vi "Coverage Analyzer View.vi"(8 "error in (no error)":errorcluster, 11 "Code Coverage":map{path, dbl}(c390)) -> (0 "error out":errorcluster)   [LabVIEW 2020, in "Coverage Analyzer.lvclass"]
uses:
  Coverage Analyzer.lvclass
  Coverage Analyzer.lvclass/Coverage Analyzer.ctl
  <vilib>/Analysis/baseanly.llb/Mean (DBL).vi
  fde09a69-7451-4da4-9368-3dcb0be6c936.vi
  <vilib>/Comparison/Less/Less Functor/Less Functor.lvclass
  <vilib>/Analysis/NI_AALBase.lvlib
panel:
  in  "Method Test Times":i32(listbox)
  out "Debug disabled VIs":string
  out "Coverage for Executed VIs":string
  out "Fraction of VIs Executed":string
  in  "Hide VIs not executed?":bool=TRUE
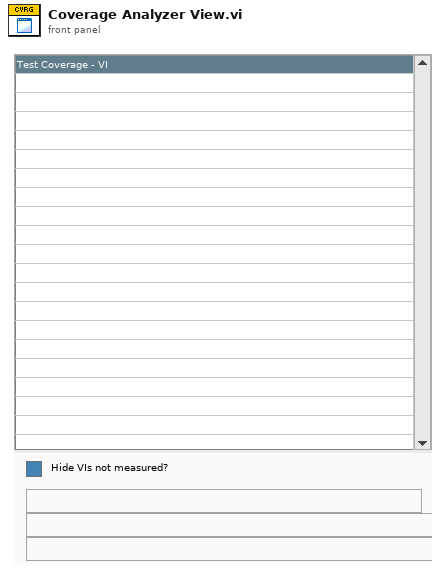
[diagram p1: front panel]
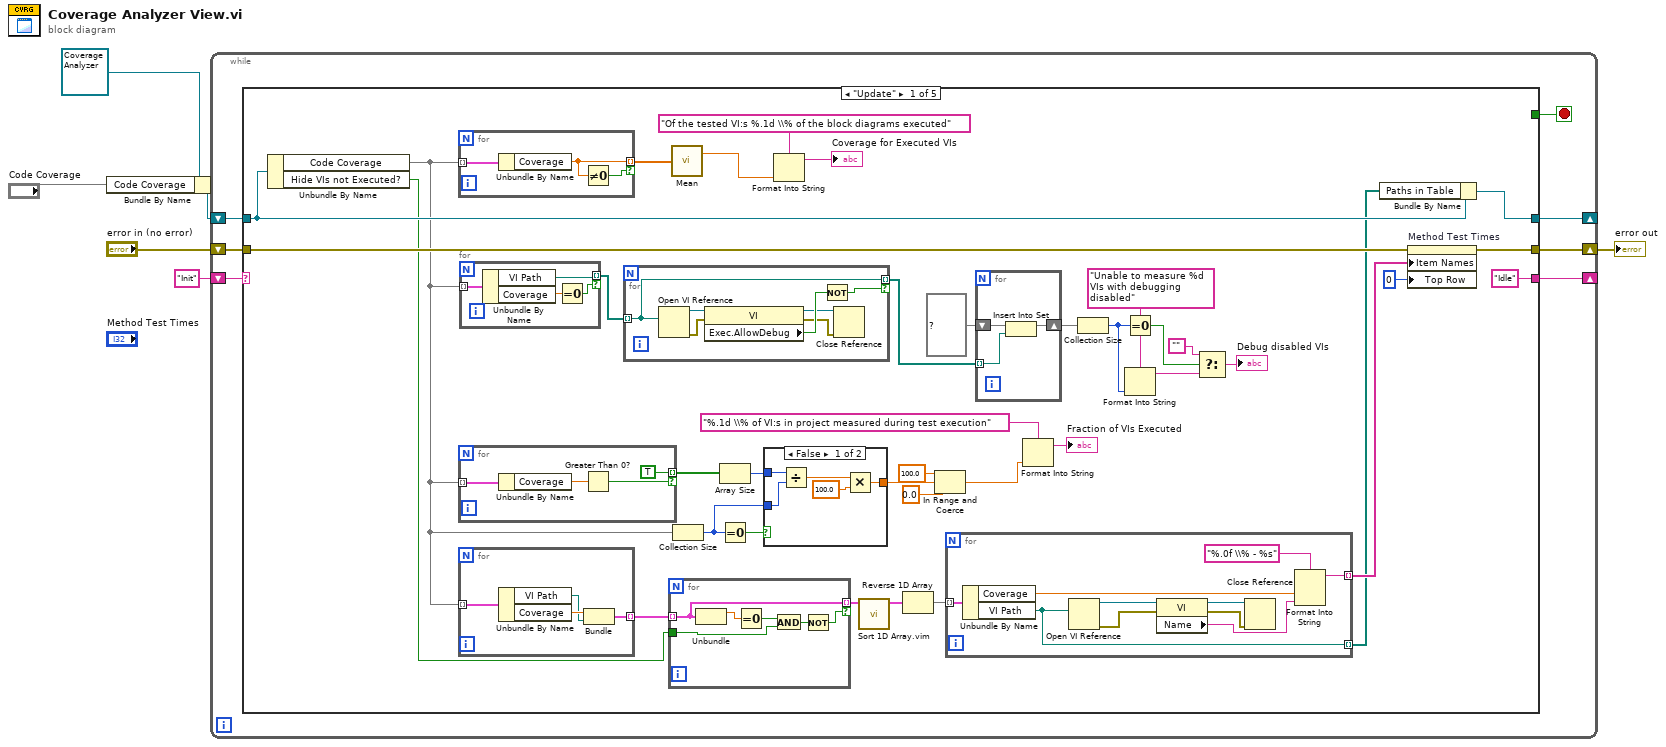
[diagram p0: block diagram]
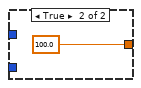
[diagram p2: hidden frame]
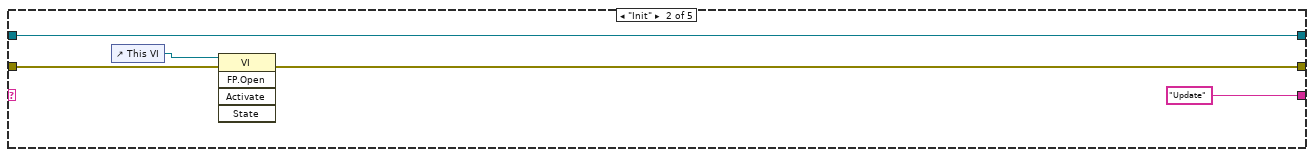
[diagram p3: hidden frame]
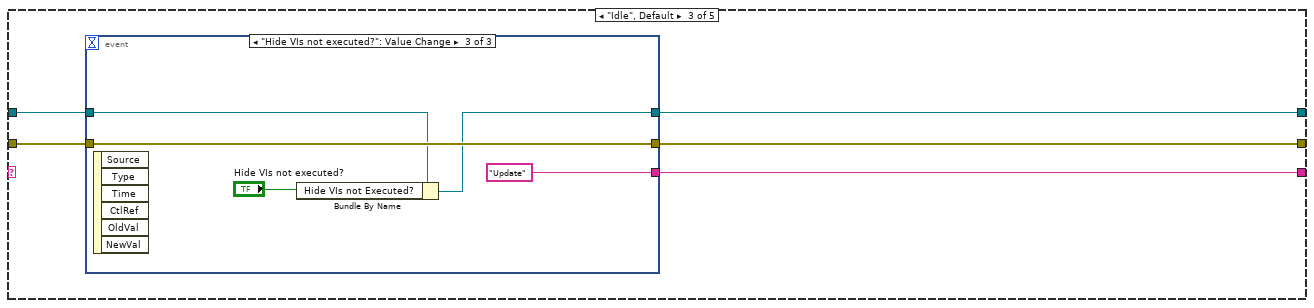
[diagram p4: hidden frame]
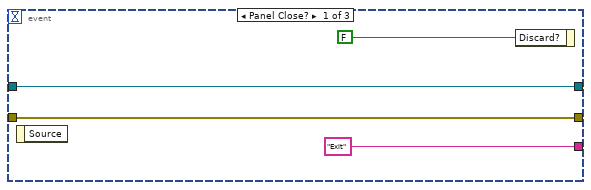
[diagram p5: hidden frame]
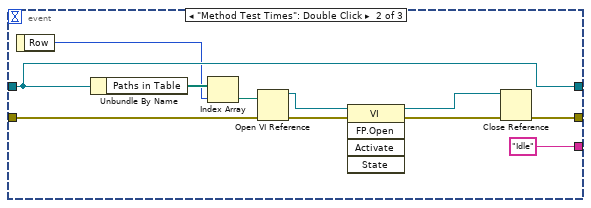
[diagram p6: hidden frame]
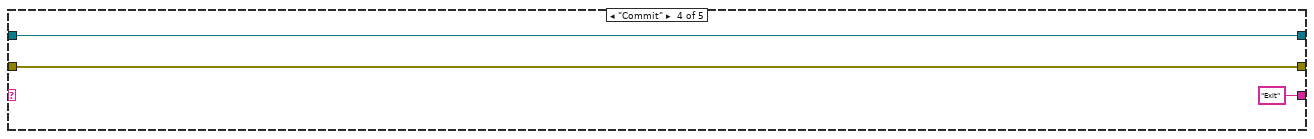
[diagram p7: hidden frame]
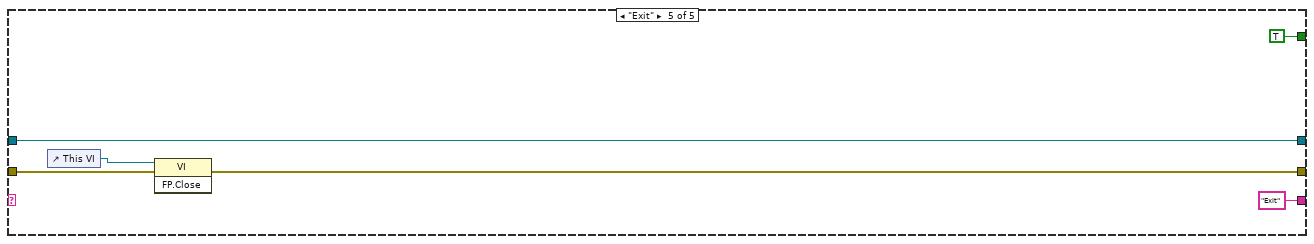
[diagram p8: hidden frame]
diagram:
  n1 = Bundle By Name(cluster=refnum<class "Coverage Analyzer.lvclass"> refnum ("Coverage Analyzer Result View.lvclass"), "Code Coverage"="Code Coverage") -> (w2:refnum<class "Coverage Analyzer.lvclass">)
  n2 = while {
    shift-right: [w10] -> _
    shift-left: w2 -> [w11]
    shift-right: [w7] -> w4
    shift-left: "error in (no error)" -> [w12]
    shift-right: [w9] -> _
    shift-left: "Init" -> [w13]
    stop <- w8 stop-if-true
    n3 = case shown="\"Update\"" w13 {
      tunnel: [w50 w101 w108 w131 w133] -> w7
      tunnel: w12 -> [w46 w100 w107 w131 w132]
      tunnel: w11 -> [w43 w99 w106 w130 w137]
      tunnel: [w48 w99 w105 w130 w137] -> w10
      tunnel: ["Idle" "Update" w104 "Exit" "Exit"] -> w9
      tunnel: [_ _ _ _ TRUE] -> w8
      frame "Update" {
        n4 = Unbundle By Name(w43) -> ("Code Coverage"=w18:map{path, dbl}, "Hide VIs not Executed?"=w17:bool)
        n5 = for {
          tunnel: w18 -> [w68] mode=indexing
          tunnel: [w67] -> w29 mode=indexing if=w66
          n6 = Unbundle By Name(w68) -> ("Coverage"=w67:dbl)
          n7 = Not Equal To 0?(x=w67) -> (x != 0?=w66:bool)
        }
        n8 = for {
          tunnel: w18 -> [w72] mode=indexing
          tunnel: [TRUE] -> w35 mode=indexing if=w69
          n9 = Unbundle By Name(w72) -> ("Coverage"=w71:dbl)
          n10 = Greater Than 0?(x=w71) -> (x > 0?=w69:bool)
        }
        n11 = for {
          tunnel: w18 -> [w88] mode=indexing
          tunnel: [w86] -> w40 mode=indexing
          n12 = Unbundle By Name(w88) -> ("VI Path"=w85:path, "Coverage"=w87:dbl)
          n13 = Bundle("Coverage"=w87, "VI Path"=w85) -> (w86:cluster{"Coverage":dbl, "VI Path":path})  [unwired: 1 in]
        }
        n14 = for {
          tunnel: w18 -> [w65] mode=indexing
          tunnel: [w62] -> w19 mode=indexing if=w63
          n15 = Unbundle By Name(w65) -> ("VI Path"=w62:path, "Coverage"=w64:dbl)
          n16 = Equal To 0?(x=w64) -> (x = 0?=w63:bool)
        }
        n17 = for {
          tunnel: w19 -> [w56] mode=indexing
          tunnel: [w56] -> w21 mode=indexing if=w55
          n18 = Open VI Reference(vi path=w56) -> (vi reference=w61:refnum<vi>, error out=w60:errorcluster)  [unwired: 5 in]
          n19 = property class="VI"(reference=w61, error in=w60) -> (reference out=w57:refnum<vi>, error out=w58:errorcluster, "Exec.AllowDebug"=w59:bool)
          n20 = Not(x=w59) -> (.not. x?=w55:bool)
          n21 = Close Reference(reference=w57, error in (no error)=w58) -> ()  [unwired: 1 out]
        }
        n22 = for {
          tunnel: [w84] -> w41 mode=indexing if=w79
          tunnel: w40 -> [w84] mode=indexing
          tunnel: w17 -> [w81]
          n23 = Unbundle(w84) -> ("Coverage"=w83:dbl)  [unwired: 1 out]
          n24 = Equal To 0?(x=w83) -> (x = 0?=w82:bool)
          n25 = And(x=w82, y=w81) -> (x .and. y?=w80:bool)
          n26 = Not(x=w80) -> (.not. x?=w79:bool)
        }
        n27 = call-poly <vilib>:"Mean.vi"("X"=w29) -> ("mean"=w30:dbl)  [unwired: 1 out]
        n28 = Collection Size(1:w18) -> (0:w33:i32)
        n29 = Array Size(array=w35) -> (size(s)=w36:i32)
        n30 = Equal To 0?(x=w33) -> (x = 0?=w32:bool)
        n31 = case shown="False" w32 {
          tunnel: w36 -> [w77 _]
          tunnel: [w74 100.0] -> w34
          tunnel: w33 -> [w75 _]
          frame False {
            n32 = Divide(x=w77, y=w75) -> (x/y=w76:dbl)
            n33 = Multiply(x=w76, y=100.0) -> (x*y=w74:dbl)
          }
          frame True {
          }
        }
        n34 = Format Into String(format string="Of the tested VI:s %.1d \\% of the block diagrams executed", w30) -> (resulting string=→"Coverage for Executed VIs":string)  [unwired: 2 in, 1 out]
        n35 = call "Sort 1D Array.vim"("unsorted array"=w41) -> ("sorted array"=w37:cluster{"Coverage":dbl, "VI Path":path}[])  [unwired: 10 in]
        n36 = Reverse 1D Array(array=w37) -> (reversed array=w38:cluster{"Coverage":dbl, "VI Path":path}[])
        n37 = In Range and Coerce(upper limit=100.0, x=w34, lower limit=0.0) -> (coerced(x)=w16:dbl)  [unwired: 1 out]
        n38 = for {
          tunnel: w38 -> [w98] mode=indexing
          tunnel: [w95] -> w49 mode=indexing
          tunnel: [w90] -> w39 mode=indexing
          n39 = Unbundle By Name(w98) -> ("Coverage"=w96:dbl, "VI Path"=w90:path)
          n40 = Open VI Reference(vi path=w90) -> (vi reference=w94:refnum<vi>, error out=w93:errorcluster)  [unwired: 5 in]
          n41 = property class="VI"(reference=w94, error in=w93) -> (reference out=w92:refnum<vi>, error out=w91:errorcluster, "Name"=w89:string)
          n42 = Close Reference(reference=w92, error in (no error)=w91) -> ()  [unwired: 1 out]
          n43 = Format Into String(format string="%.0f \\% - %s", w96, w89) -> (resulting string=w95:string)  [unwired: 2 in, 1 out]
        }
        n44 = for {
          shift-right: [w53] -> w23
          shift-left: set{path} {} ("VIs") -> [w54]
          tunnel: w21 -> [w52] mode=indexing
          n45 = Insert Into Set(10:w52, 11:w54) -> (3:w53:set{path})  [unwired: 1 out]
        }
        n46 = Format Into String(format string="%.1d \\% of VI:s in project measured during test execution", w16) -> (resulting string=→"Fraction of VIs Executed":string)  [unwired: 2 in, 1 out]
        n47 = Collection Size(1:w23) -> (0:w25:i32)
        n48 = Equal To 0?(x=w25) -> (x = 0?=w24:bool)
        n49 = Format Into String(format string="Unable to measure %d VIs with debugging disabled", w25) -> (resulting string=w26:string)  [unwired: 2 in, 1 out]
        n50 = Select(t="", s=w24, f=w26) -> (s? t:f=→"Debug disabled VIs":string)
        n51 = Bundle By Name(cluster=w43, "Paths in Table"=w39) -> (w48:refnum<class "Coverage Analyzer.lvclass">)
        n52 = property on="Method Test Times" class="LstBox (strict)"(error in=w46, "Item Names"=w49, "Top Row"=0) -> (error out=w50:errorcluster)  [unwired: 1 in, 1 out]
      }
      frame "Init" {
        n53 = control-ref of="This VI"() -> (w102:refnum<vi>)
        n54 = invoke class="VI" method="FP.Open"(reference=w102, error in=w100) -> (error out=w101:errorcluster)  [unwired: 3 in, 4 out]
      }
      frame "Idle", Default {
        n55 = event shown="[2] \"Hide VIs not executed?\": Value Change" {
          selector: _ -> [_ _ _]
          dyn-events: _ -> [_ _ _]
          timeout: _ -> [_ _ _]
          tunnel: [w112 w114 w128] -> w108
          tunnel: w107 -> [w112 w113 w128]
          tunnel: w106 -> [w111 w122 w127]
          tunnel: [w111 w122 w125] -> w105
          tunnel: ["Exit" "Idle" "Update"] -> w104
          event Panel Close? {
            n56 = event-data() -> ()  [unwired: 1 in, 1 out]
            n57 = event-data("Discard?"=FALSE) -> ()  [unwired: 1 in, 1 out]
          }
          event "Method Test Times": Double Click {
            n58 = event-data() -> ("Row"=w120:i32)  [unwired: 1 in]
            n59 = Unbundle By Name(w122) -> ("Paths in Table"=w121:path[])
            n60 = Index Array(array=w121, index=w120) -> (element=w119:path)
            n61 = Open VI Reference(vi path=w119, error in (no error)=w113) -> (vi reference=w118:refnum<vi>, error out=w117:errorcluster)  [unwired: 4 in]
            n62 = invoke class="VI" method="FP.Open"(reference=w118, error in=w117) -> (reference out=w116:refnum<vi>, error out=w115:errorcluster)  [unwired: 3 in, 3 out]
            n63 = Close Reference(reference=w116, error in (no error)=w115) -> (error out=w114:errorcluster)
          }
          event "Hide VIs not executed?": Value Change {
            n64 = event-data() -> ()  [unwired: 1 in, 6 out]
            n65 = Bundle By Name(cluster=w127, "Hide VIs not Executed?"="Hide VIs not executed?") -> (w125:refnum<class "Coverage Analyzer.lvclass">)
          }
        }
      }
      frame "Commit" {
      }
      frame "Exit" {
        n66 = control-ref of="This VI"() -> (w134:refnum<vi>)
        n67 = invoke class="VI" method="FP.Close"(reference=w134, error in=w132) -> (error out=w133:errorcluster)  [unwired: 1 in, 2 out]
      }
    }
  }
  "error out" <- w4
